vi "Convert I16x16 to U256.vi"(7 "I16x16 Data":i16[](array[numeric])=[0, 0, 0, 0, 0, 0, 0, 0, 0, 0, 0, 0, 0, 0, 0, 0]) -> (8 "U64x4 CLuster":T1)   [LabVIEW 2012]
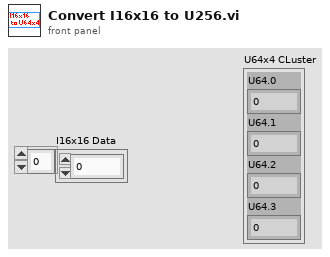
[diagram p1: front panel]
types:
  T1 = cluster{"U64.0":u64, "U64.1":u64, "U64.2":u64, "U64.3":u64}
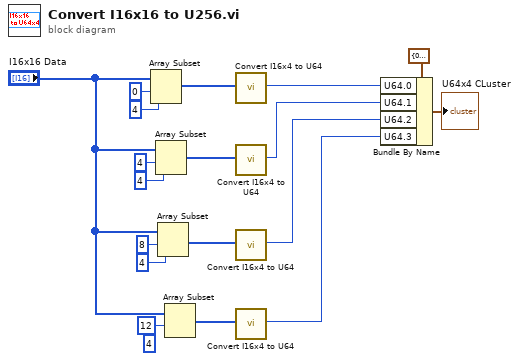
[diagram p0: block diagram]
diagram:
  (unwired) 4 ("length")
  n1 = Array Subset(array="I16x16 Data", index=0, length=4) -> (w10:i16[])
  n2 = Array Subset(array="I16x16 Data", index=4, length=4) -> (w9:i16[])
  n3 = Array Subset(array="I16x16 Data", index=8, length=4) -> (w8:i16[])
  n4 = Array Subset(array="I16x16 Data", index=12) -> (w7:i16[])  [unwired: 1 in]
  n5 = call <userlib>:"Convert I16x4 to U64.vi"("Input Data"=w10) -> ("U64"=w5:u64)  [unwired: 18 in]
  n6 = call <userlib>:"Convert I16x4 to U64.vi"("Input Data"=w9) -> ("U64"=w4:u64)  [unwired: 18 in]
  n7 = call <userlib>:"Convert I16x4 to U64.vi"("Input Data"=w8) -> ("U64"=w3:u64)  [unwired: 18 in]
  n8 = call <userlib>:"Convert I16x4 to U64.vi"("Input Data"=w7) -> ("U64"=w2:u64)  [unwired: 18 in]
  n9 = Bundle By Name(cluster=T1 {"U64.0"=0, "U64.1"=0, "U64.2"=0, "U64.3"=0} ("Output Data"), "U64.0"=w5, "U64.1"=w4, "U64.2"=w3, "U64.3"=w2) -> (→"U64x4 CLuster":T1)
